vi "niFpga wdp fft pfft dummy.vi"(6 "enable":bool, 11 "data in":T2(array[cluster])=[{"data re"=0.0, "data im"=0.0}, {"data re"=0.0, "data im"=0.0}]) -> (3 "data out":T1(array[cluster]))   [LabVIEW 2017]
types:
  T1 = cluster{"x-y":fxp<+/-,20,13>, "x-y":fxp<+/-,20,13>}[]
  T2 = cluster{"data re":fxp<+/-,19,12>, "data im":fxp<+/-,19,12>}[]
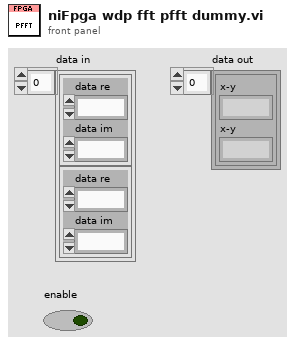
[diagram p1: front panel]
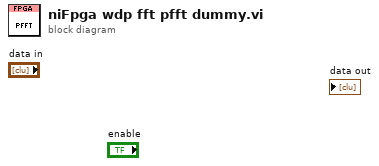
[diagram p0: block diagram]
diagram:
